vi "closeTestLog.vi"(8 "error in (no error)":errorcluster, 11 "Model in":refnum<class "Model.lvclass">) -> (0 "error out":errorcluster, 3 "Model out":refnum<class "Model.lvclass">)   [LabVIEW 2015, in "Model.lvclass"]
uses:
  Model.lvclass
  Model.lvclass/Model.ctl
  TestLog/ITestLog/ITestLog.lvclass
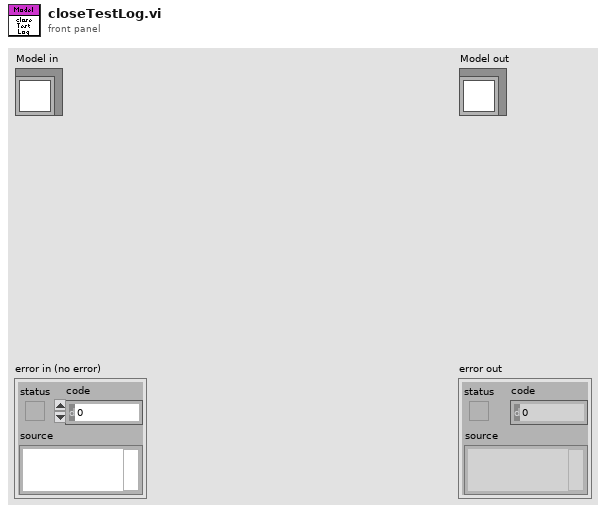
[diagram p1: front panel]
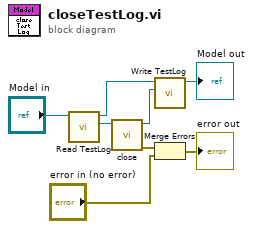
[diagram p0: block diagram]
diagram:
  n1 = call "Read TestLog.vi"("Model in"="Model in") -> ("ITestLog.lvclass"=w7:refnum<class "ITestLog.lvclass">, "Model out"=w6:refnum<class "Model.lvclass">)  [unwired: 9 in]
  n2 = call-dynamic "close.vi"("ITestLog in"=w7) -> ("error out"=w3:errorcluster, "ITestLog out"=w8:refnum<class "ITestLog.lvclass">)  [unwired: 9 in]
  n3 = call "Write TestLog.vi"("ITestLog.lvclass"=w8, "Model in"=w6) -> ("Model out"=→"Model out":refnum<class "Model.lvclass">)  [unwired: 9 in]
  n4 = Merge Errors(w3, "error in (no error)") -> (→"error out":errorcluster)
